vi "RSZVB Get IMOD Lower Tone Source.vi"(8 "error in (no error)":errorcluster {"code" format="%.0x"}, 10 "Channel (1)":i32=1, 11 "VISA session":refnum<visa-resource-name>) -> (0 "error out":errorcluster {"code" format="%.0x"}, 1 "Source":i32, 3 "dup VISA session":refnum<visa-resource-name>, 5 "Source Number":i32)   [LabVIEW 2011]
doc: "This VI returns the source for the lower tone signal that is used for the intermodulation measurement.\n\nNote(s):\n\n(1) This VI is not available for R&S ZVB instrument.\n\nRemote-control command(s):\n[SENSe<Ch>:]FREQuency:IMODulation:LTONe?"
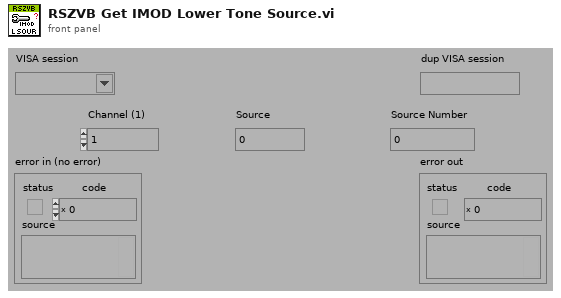
[diagram p1: front panel]
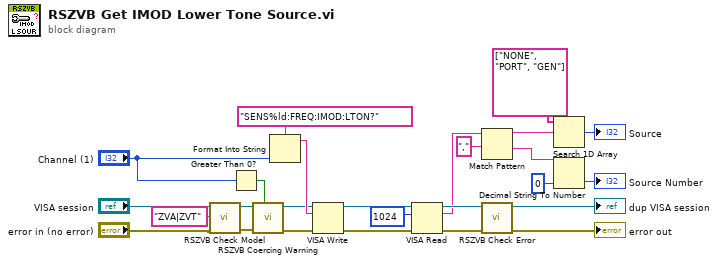
[diagram p0: block diagram]
diagram:
  n1 = call "RSZVB Check Model.vi"("error in (no error)"="error in (no error)", "Model"="ZVA|ZVT", "VISA session"="VISA session") -> ("error out"=w2:errorcluster, "dup VISA session"=w1:refnum<visa-resource-name>)  [unwired: 7 in]
  n2 = Greater Than 0?(x="Channel (1)") -> (x > 0?=w24:bool)
  n3 = call "RSZVB Coercing Warning.vi"("In Range?"=w24, "error in (no error)"=w2, "VISA session"=w1) -> ("error out"=w21:errorcluster, "dup VISA session"=w22:refnum<visa-resource-name>)  [unwired: 7 in]
  n4 = Format Into String(format string="SENS%ld:FREQ:IMOD:LTON?", "Channel (1)") -> (resulting string=w23:string)  [unwired: 2 in, 1 out]
  n5 = VISA Write(VISA resource name=w22, write buffer=w23, error in (no error)=w21) -> (VISA resource name out=w20:refnum<visa-resource-name>, error out=w19:errorcluster)  [unwired: 1 out]
  n6 = VISA Read(VISA resource name=w20, byte count=u32 1024 ("byte count (0)"), error in (no error)=w19) -> (VISA resource name out=w17:refnum<visa-resource-name>, read buffer=w6:string, error out=w16:errorcluster)  [unwired: 1 out]
  n7 = Match Pattern(string=w6, regular expression="," ("search string/char (-)")) -> (before substring=w12:string, after substring=w9:string)  [unwired: 1 in, 2 out]
  n8 = call "RSZVB Check Error.vi"("error in (no error)"=w16, "VISA session"=w17) -> ("error out"=→"error out":errorcluster, "dup VISA session"=→"dup VISA session":refnum<visa-resource-name>)  [unwired: 8 in]
  n9 = Search 1D Array(1D array=string[] ["NONE", "PORT", "GEN"], element=w12) -> (index of element=→"Source":i32)  [unwired: 1 in]
  n10 = Decimal String To Number(string=w9, default (0L)=0) -> (number=→"Source Number":i32)  [unwired: 1 in, 1 out]
